vi "Run.vi"(8 "error in":errorcluster, 10 "Execution Plan":T1={"Exe Path"=path "", "Args"=[], "Timeout"=-1}, 11 "Process Executor in":refnum<class "Process Executor.lvclass">) -> (0 "error out":errorcluster, 3 "Process Executor out":refnum<class "Process Executor.lvclass">)   [LabVIEW 2025, in "Process Executor.lvclass"]
doc: "Launches an external executable with arguments and manages its execution timeout."
uses:
  Process Executor.lvclass
  Type Definitions/Execution Plan--cluster.ctl
  <userlib>/_OpenG.lib/file/file.llb/File Exists - Scalar__ogtk.vi
  <userlib>/_OpenG.lib/file/file.llb/Strip Path Extension - Path__ogtk.vi
  <userlib>/_OpenG.lib/file/file.llb/openg_file.lvlib
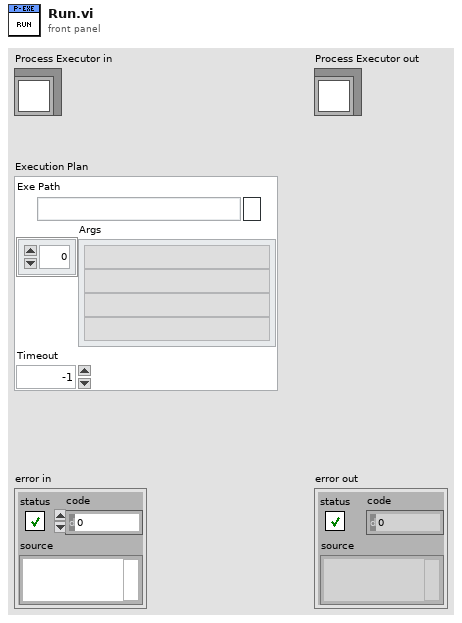
[diagram p1: front panel]
types:
  T1 = typedef "Execution Plan--cluster.ctl" = cluster{"Exe Path":path, "Args":string[], "Timeout":i32}
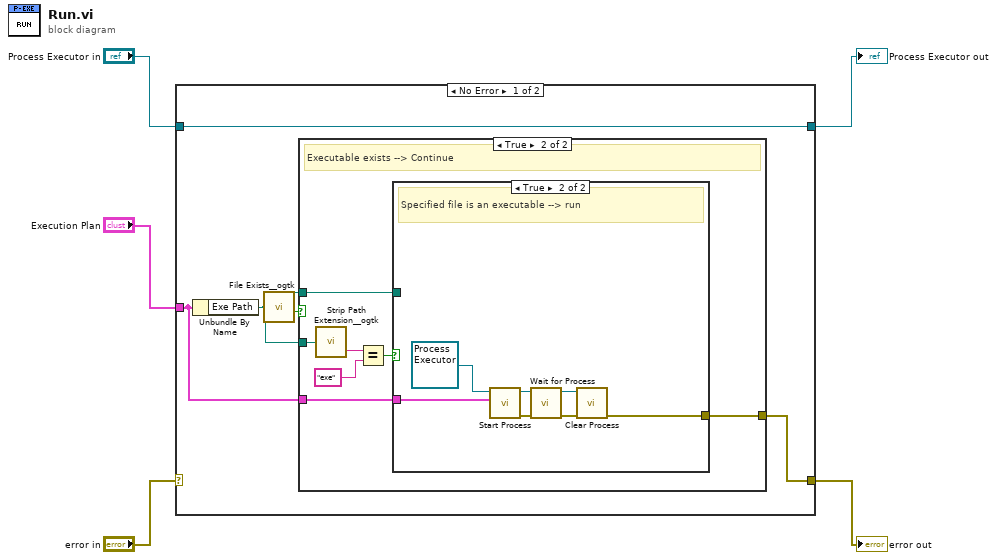
[diagram p0: block diagram]
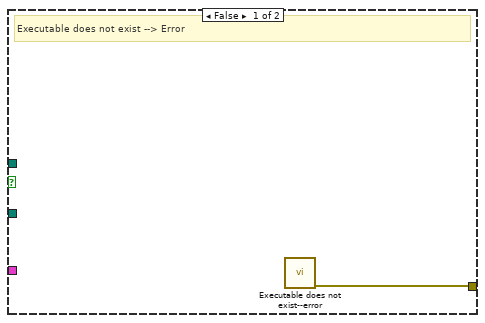
[diagram p2: hidden frame]
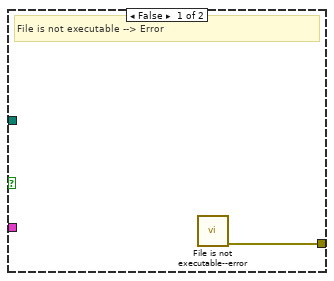
[diagram p3: hidden frame]
diagram:
  n1 = case shown="No Error" "error in" {
    selector: "error in" -> [_ w28]
    tunnel: [w10 w28] -> w4
    tunnel: "Execution Plan" -> [w8 _]
    tunnel: "Process Executor in" -> [w6 w27]
    tunnel: [w6 w27] -> w1
    frame No Error {
      n2 = Unbundle By Name(w8) -> ("Exe Path"=w7:path)
      n3 = call-poly <userlib>:"File Exists__ogtk.vi"("file path"=w7) -> ("exists"=w9:bool)  [unwired: 6 in, 1 out]
      n4 = case shown="True" w9 {
        tunnel: [w11 w18] -> w10
        tunnel: w7 -> [_ w17]
        tunnel: w8 -> [_ w13]
        tunnel: w7 -> [_ w12]
        frame False {
          # "Executable does not exist --> Error"
          n5 = call "Executable does not exist--error.vi"() -> ("error out"=w11:errorcluster)  [unwired: 11 in]
        }
        frame True {
          # "Executable exists --> Continue"
          n6 = call-poly <userlib>:"Strip Path Extension__ogtk.vi"("path"=w17) -> ("extension"=w16:string)  [unwired: 1 out]
          n7 = Equal?(x=w16, y="exe") -> (x = y?=w14:bool)
          n8 = case shown="True" w14 {
            tunnel: [w19 w24] -> w18
            tunnel: w13 -> [_ w23]
            tunnel: w12 -> [_ _]
            frame False {
              # "File is not executable --> Error"
              n9 = call "File is not executable--error.vi"() -> ("error out"=w19:errorcluster)  [unwired: 11 in]
            }
            frame True {
              # "Specified file is an executable --> run"
              n10 = call "Start Process.vi"("Execution Plan"=w23, "Process Executor in"=refnum<class "Process Executor.lvclass"> refnum) -> ("error out"=w26:errorcluster, "Process Executor out"=w21:refnum<class "Process Executor.lvclass">)  [unwired: 8 in]
              n11 = call "Wait for Process.vi"("error in"=w26, "Process Executor in"=w21) -> ("error out"=w25:errorcluster, "Process Executor out"=w20:refnum<class "Process Executor.lvclass">)  [unwired: 8 in]
              n12 = call "Clear Process.vi"("error in (no error)"=w25, "Process Executor in"=w20) -> ("error out"=w24:errorcluster)  [unwired: 8 in, 1 out]
            }
          }
        }
      }
    }
    frame Error {
      # "Pass error without further action"
    }
  }
  "error out" <- w4
  "Process Executor out" <- w1
